vi "Pick Best Object Layout Class.vi"(7 "application reference":refnum<vi>, 8 "error in":errorcluster, 10 "rescan classes (F)":bool, 11 "GObj Refnum":refnum<vi>) -> (0 "error out":errorcluster, 2 "found?":bool, 3 "object layout class":refnum<class "Object Layout.lvclass">)   [LabVIEW 2010, in "NI_SE_Front Panel Layout.lvlib"]
uses:
  NI_SE_Front Panel Layout.lvlib
  Object Layout Classes/Object Layout/Object Layout.lvclass
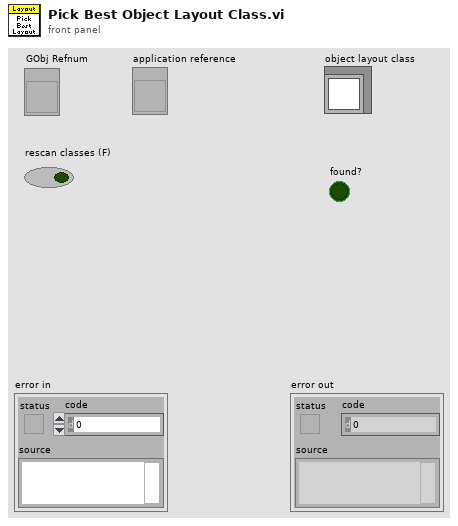
[diagram p1: front panel]
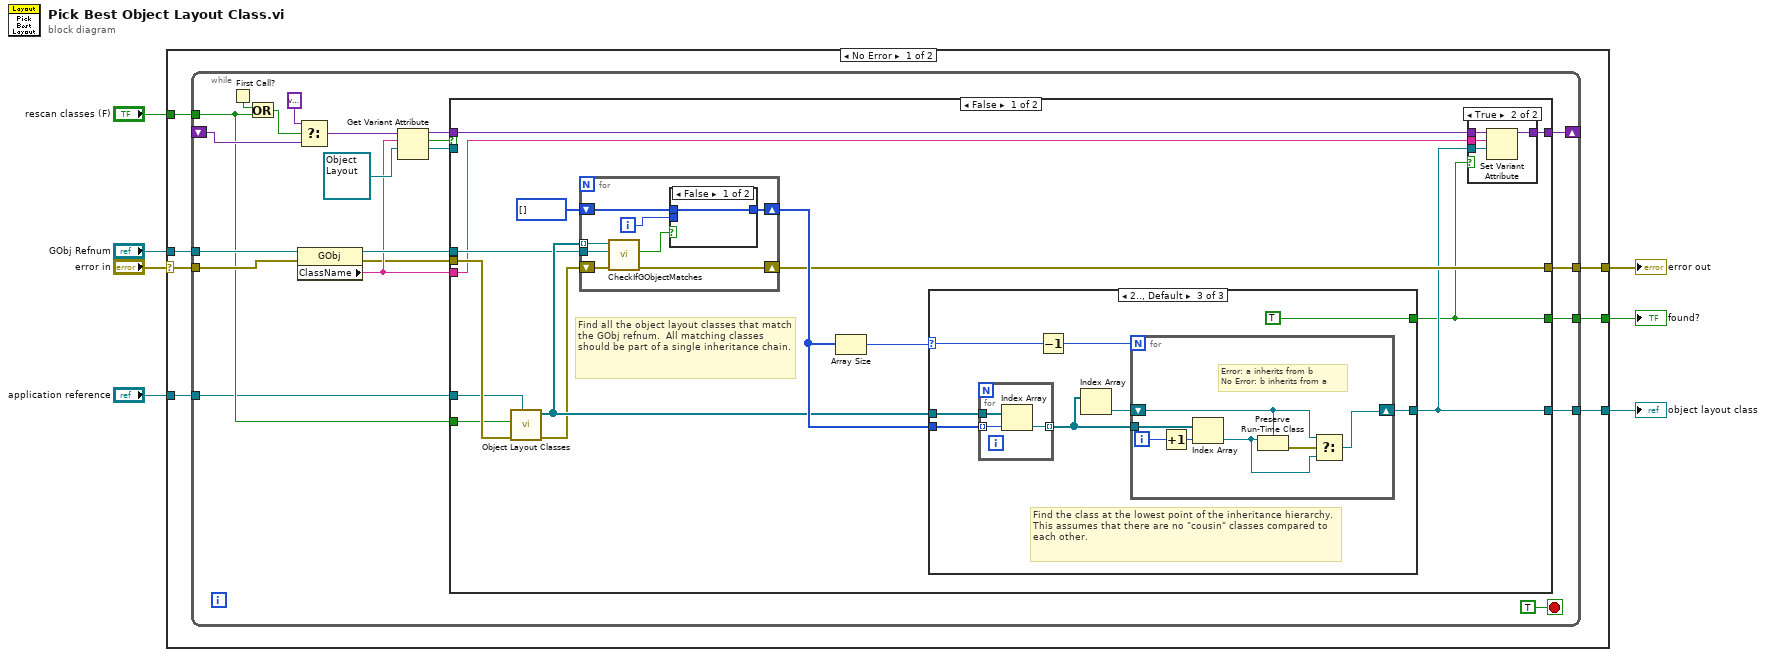
[diagram p0: block diagram]
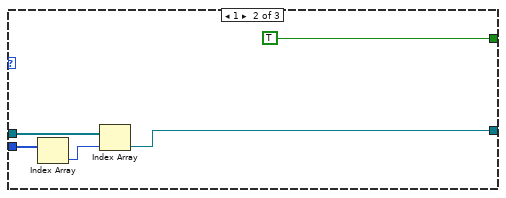
[diagram p4: hidden frame]
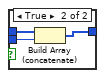
[diagram p5: hidden frame]
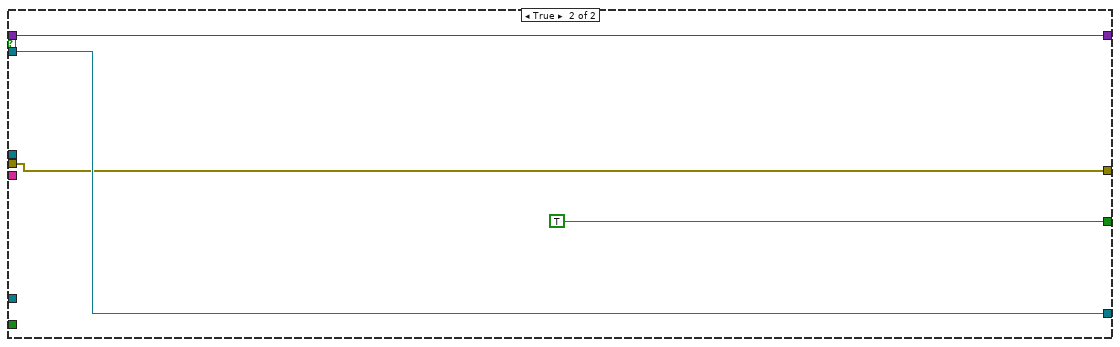
[diagram p6: hidden frame]
diagram:
  n1 = case shown="No Error" "error in" {
    selector: "error in" -> [w11 w95]
    tunnel: [w12 w95] -> w6
    tunnel: "GObj Refnum" -> [w14 _]
    tunnel: [w10 _] -> w4
    tunnel: [w13 _] -> w3
    tunnel: "rescan classes (F)" -> [w9 _]
    tunnel: "application reference" -> [w8 _]
    frame No Error {
      n2 = while {
        tunnel: w14 -> [w29]
        tunnel: [w35] -> w13
        tunnel: [w34] -> w12
        tunnel: w11 -> [w27]
        tunnel: [w33] -> w10
        shift-right: [w21] -> _
        shift-left: _ -> [w30]
        tunnel: w9 -> [w16]
        tunnel: w8 -> [w15]
        stop <- TRUE stop-if-true
        n3 = First Call?() -> (First Call?: T/F=w18:bool)
        n4 = Or(x=w18, y=w16) -> (x .or. y?=w17:bool)
        n5 = property class="GObj"(reference=w29, error in=w27) -> (reference out=w28:refnum<vi>, error out=w19:errorcluster, "ClassName"=w20:string)
        n6 = Select(t=variant ("Variant"), s=w17, f=w30) -> (s? t:f=w26:variant)
        n7 = Get Variant Attribute(Variant=w26, name=w20, default value (empty Variant)=refnum<class "Object Layout.lvclass"> refnum ("NI_SE_Front Panel Layout.lvlib:Object Layout.lvclass")) -> (duplicate Variant=w23:variant, found=w24:bool, value=w22:refnum<class "Object Layout.lvclass">)  [unwired: 1 in, 1 out]
        n8 = case shown="False" w24 {
          tunnel: [w40 w94] -> w35
          tunnel: [w48 w93] -> w34
          tunnel: [w38 TRUE] -> w33
          tunnel: w28 -> [w44 _]
          tunnel: w19 -> [w43 w93]
          tunnel: w23 -> [w42 w91]
          tunnel: w22 -> [_ w94]
          tunnel: [w41 w91] -> w21
          tunnel: w20 -> [w39 _]
          tunnel: w16 -> [w37 _]
          tunnel: w15 -> [w36 _]
          frame False {
            # "Find all the object layout classes that match the GObj refnum.  All matching classes should be part of a single inheritance chain."
            n9 = call "Object Layout Classes.vi"("application reference"=w36, "error in"=w43, "rescan (F)"=w37) -> ("error out"=w47:errorcluster, "object layout classes"=w49:refnum<class "Object Layout.lvclass">[])  [unwired: 7 in]
            n10 = for {
              tunnel: w49 -> [w82] mode=indexing
              tunnel: w44 -> [w86]
              shift-right: [w84] -> w48
              shift-left: w47 -> [w85]
              shift-right: [w79] -> w50
              shift-left: i32[] [] ("Array") -> [w80]
              i -> [w81]
              n11 = call-dynamic "CheckIfGObjectMatches.vi"("error in (no error)"=w85, "GObj Refnum"=w86, "Object Layout in"=w82) -> ("error out"=w84:errorcluster, "compatible?"=w83:bool)  [unwired: 7 in]
              n12 = case shown="False" w83 {
                tunnel: w80 -> [w87 w89]
                tunnel: w81 -> [_ w88]
                tunnel: [w87 w90] -> w79
                frame False {
                }
                frame True {
                  n13 = Build Array (concatenate)(w89, w88) -> (w90:i32[])
                }
              }
            }
            n14 = Array Size(array=w50) -> (size(s)=w46:i32)
            n15 = case shown="2.., Default" w46 {
              selector: w46 -> [_ _ w65]
              tunnel: w50 -> [_ w60 w68]
              tunnel: [_ w57 w66] -> w40
              tunnel: w49 -> [_ w59 w67]
              tunnel: [_ TRUE TRUE] -> w38
              frame 0 {
                # "No matches found"
              }
              frame 1 {
                n16 = Index Array(array=w60) -> (element=w58:i32)  [unwired: 1 in]
                n17 = Index Array(array=w59, index=w58) -> (element=w57:refnum<class "Object Layout.lvclass">)
              }
              frame 2.., Default {
                # "Find the class at the lowest point of the inheritance hierarchy.  This assumes that there are no \"cousin\" classes compared to each other."
                n18 = for {
                  tunnel: w67 -> [w78]
                  tunnel: w68 -> [w77] mode=indexing
                  tunnel: [w76] -> w63 mode=indexing
                  n19 = Index Array(array=w78, index=w77) -> (element=w76:refnum<class "Object Layout.lvclass">)
                }
                n20 = Decrement(x=w65) -> (x-1=w64:i32)
                n21 = Index Array(array=w63) -> (element=w62:refnum<class "Object Layout.lvclass">)  [unwired: 1 in]
                n22 = for {
                  N: w64 -> [_]
                  tunnel: w63 -> [w75]
                  shift-right: [w69] -> w66
                  shift-left: w62 -> [w71]
                  i -> [w74]
                  # "Error: a inherits from b\nNo Error: b inherits from a"
                  n23 = Increment(x=w74) -> (x+1=w73:i32)
                  n24 = Index Array(array=w75, index=w73) -> (element=w70:refnum<class "Object Layout.lvclass">)
                  n25 = Preserve Run-Time Class(object in=w70, 2:w71) -> (error out=w72:errorcluster)  [unwired: 1 in, 1 out]
                  n26 = Select(t=w71, s=w72, f=w70) -> (s? t:f=w69:refnum<class "Object Layout.lvclass">)
                }
              }
            }
            n27 = case shown="True" w38 {
              tunnel: w42 -> [w51 w55]
              tunnel: [w51 w54] -> w41
              tunnel: w40 -> [_ w53]
              tunnel: w39 -> [_ w52]
              frame False {
              }
              frame True {
                n28 = Set Variant Attribute(Variant=w55, name=w52, value=w53) -> (Variant out=w54:variant)  [unwired: 1 in, 2 out]
              }
            }
          }
          frame True {
          }
        }
      }
    }
    frame Error {
    }
  }
  "error out" <- w6
  "found?" <- w4
  "object layout class" <- w3
